vi "GetType.vi"(8 "error in (no error)":errorcluster, 11 "Configure NofRecords Msg":refnum<class "Configure NofRecords Msg.lvclass">) -> (0 "error out":errorcluster, 2 "Data Sample":variant, 3 "Configure NofRecords Msg":refnum<class "Configure NofRecords Msg.lvclass">)   [LabVIEW 2015, in "CS++MCS.lvlib" / "Configure NofRecords Msg.lvclass"]
uses:
  Configure NofRecords Msg.lvclass
  Configure NofRecords Msg.lvclass/Configure NofRecords Msg.ctl
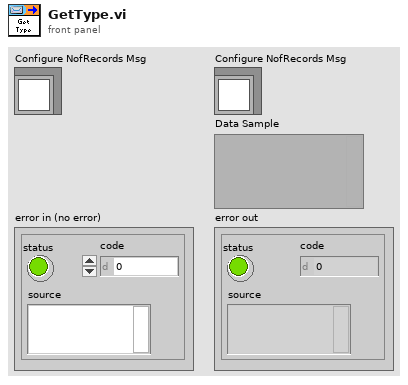
[diagram p1: front panel]
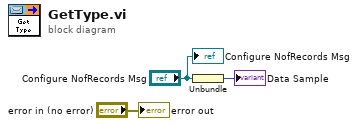
[diagram p0: block diagram]
diagram:
  n1 = Unbundle("Configure NofRecords Msg") -> (→"Data Sample":i32)
  "error out" <- "error in (no error)"
  "Configure NofRecords Msg" <- "Configure NofRecords Msg"
